vi "libssh2_agent_get_identity.vi"(8 "error in (no error)":errorcluster, 10 "prev":T1, 11 "agent":T2) -> (0 "error out":errorcluster, 1 "end reached":bool, 2 "store":T1)   [LabVIEW 2013, in "libssh2.lvlib"]
doc: "Gets a public key off the collection of public keys managed by ssh-agent."
uses:
  libssh2.lvlib
  Agent Refnum.ctl
  Agent Public Key Refnum.ctl
  Not A Agent.vi
  <vilib>/Utility/error.llb/Error Cluster From Error Code.vi
  Global Settings.vi
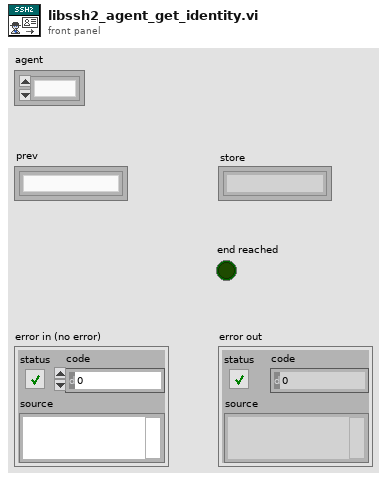
[diagram p1: front panel]
types:
  T1 = typedef "libssh2.lvlib/Agent Public Key Refnum.ctl" = refnum<k1>
  T2 = typedef "libssh2.lvlib/Agent Refnum.ctl" = refnum<k1>
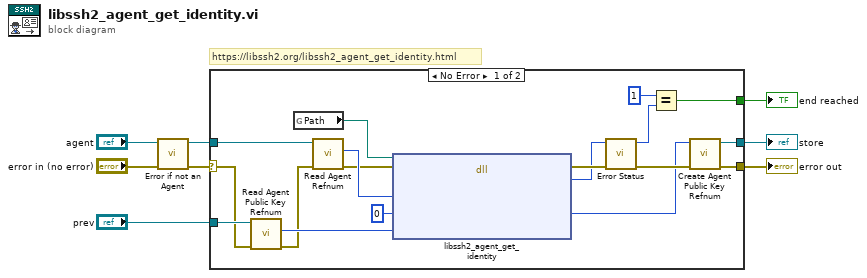
[diagram p0: block diagram]
diagram:
  # "https://libssh2.org/libssh2_agent_get_identity.html"
  n1 = call "Error if not an Agent.vi"("error in (no error)"="error in (no error)", "agent"="agent") -> ("error out"=w3:errorcluster, "agent out"=w1:T2)  [unwired: 8 in]
  n2 = case shown="No Error" w3 {
    selector: w3 -> [w11 w27]
    tunnel: w1 -> [w26 _]
    tunnel: [w25 w27] -> w8
    tunnel: [w24 _] -> w6
    tunnel: [w23 _] -> w5
    tunnel: "prev" -> [w22 _]
    frame No Error {
      n3 = call "Read Agent Public Key Refnum.vi"("error in (no error)"=w11, "agent public key"=w22) -> ("error out"=w10:errorcluster, "libssh2_agent_publickey*"=w13:u64)  [unwired: 8 in]
      n4 = global read "Global Settings.vi" "Path"() -> (w21:path)
      n5 = call "Read Agent Refnum.vi"("error in (no error)"=w10, "agent"=w26) -> ("error out"=w12:errorcluster, "LIBSSH2_AGENT*"=w20:u64)  [unwired: 8 in]
      n6 = dll-call lib="?" fn="libssh2_agent_get_identity"(path in=w21, error in=w12, "agent"=w20, "store"=u64 0, "prev"=w13) -> (error out=w17:errorcluster, "return value"=w16:i32, "store"=w14:u64)  [unwired: 3 in, 1 out]
      n7 = call "Error Status.vi"("error in (no error)"=w17, "return value"=w16) -> ("error out"=w15:errorcluster, "return value out"=w18:i32)  [unwired: 8 in]
      n8 = Equal?(x=1, y=w18) -> (x = y?=w24:bool)
      n9 = call "Create Agent Public Key Refnum.vi"("error in (no error)"=w15, "libssh2_agent_publickey*"=w14) -> ("error out"=w25:errorcluster, "agent public key"=w23:T1)  [unwired: 8 in]
    }
    frame Error {
    }
  }
  "error out" <- w8
  "end reached" <- w6
  "store" <- w5
